vi "Generate Waveform.vi"(0 "signal configuration":refnum<class "SV MLS.lvclass">, 5 "template waveform":waveform(dbl), 9 "block duration (s)":i32, 11 "error in (no error)":errorcluster) -> (4 "signal configuration":refnum<class "SV MLS.lvclass">, 6 "output waveform":waveform(dbl), 10 "samples":i32, 15 "error out":errorcluster)   [LabVIEW 2017, in "SV MLS.lvclass"]
uses:
  <vilib>/addons/_NISVFA/_Generation/Signal Generation/SV MLS/SV MLS.lvclass
  C:/Program Files (x86)/National Instruments/LabVIEW 2017/vi.lib/addons/_NISVFA/_Generation/Signal Generation/SV Signal/SV Signal.lvclass
  <vilib>/addons/_NISVFA/_Generation/Signal Generation/SV Signal/SV Signal.lvclass/SV Signal.ctl
  <vilib>/addons/_NISVFA/_Generation/Signal Generation/SV MLS/SV MLS.lvclass/SV MLS.ctl
  <vilib>/Analysis/NI_AALBase.lvlib
  <vilib>/addons/_NISVFA/_Generation/Signal Generation/SV Signal/SV Signal.lvclass
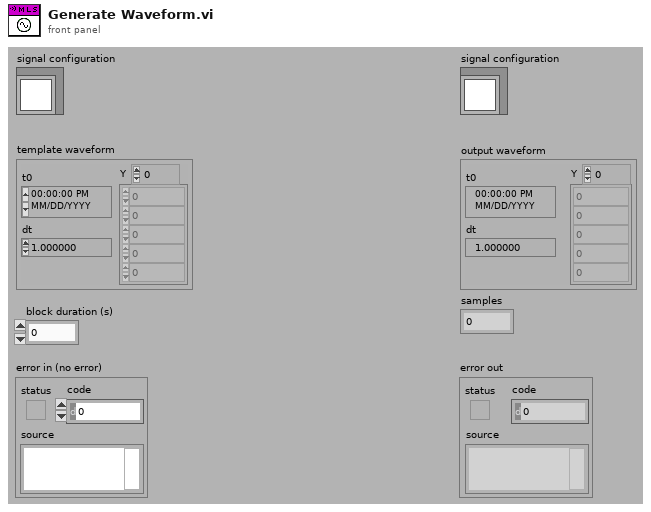
[diagram p1: front panel]
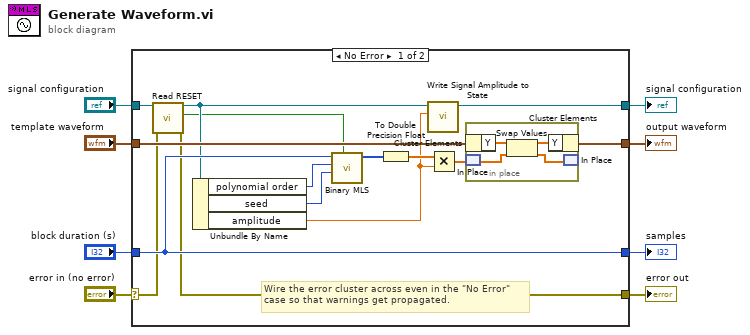
[diagram p0: block diagram]
diagram:
  n1 = case shown="No Error" "error in (no error)" {
    selector: "error in (no error)" -> [w10 w30]
    tunnel: [w9 w30] -> w7
    tunnel: [w15 w29] -> w5
    tunnel: "signal configuration" -> [w13 w29]
    tunnel: [w23 w28] -> w4
    tunnel: [w16 _] -> w3
    tunnel: "block duration (s)" -> [w16 _]
    tunnel: "template waveform" -> [w17 w28]
    frame No Error {
      # "Wire the error cluster across even in the \"No Error\"\ncase so that warnings get propagated."
      n2 = call <vilib>:"Read RESET.vi"("error in (no error)"=w10, "SV Signal in"=w13) -> ("error out"=w9:errorcluster, "RESET"=w11:bool, "SV Signal out"=w12:refnum<class "SV MLS.lvclass">)  [unwired: 7 in]
      n3 = Unbundle By Name(w12) -> ("polynomial order"=w22:i32, "seed"=w21:i64, "amplitude"=w14:dbl)
      n4 = call <vilib>:"Binary MLS.vi"("initialize?"=w11, "seed"=w21, "polynomial order"=w22, "samples"=w16) -> ("mls sequence"=w20:u8[])  [unwired: 6 in, 1 out]
      n5 = To Double Precision Float(number=w20) -> (double precision float=w19:dbl[])
      n6 = call <vilib>:"Write Signal Amplitude to State.vi"("amplitude"=w14, "SV Signal in"=w12) -> ("SV Signal out"=w15:refnum<class "SV MLS.lvclass">)  [unwired: 8 in, 1 out]
      n7 = Multiply(x=w19, y=w14) -> (x*y=w18:dbl[])
      n8 = in-place {
        n9 = in-place-cluster #1(w17) -> ("Y"=w27:dbl[])
        n10 = in-place-match #2(w18) -> (w25:dbl[])
        n11 = Swap Values(12:w27, 14:w25) -> (1:w26:dbl[], 3:w24:dbl[])  [unwired: 1 in]
        n12 = in-place-cluster #1("Y"=w26) -> (w23:waveform(dbl))
        n13 = in-place-match #2(w24) -> ()  [unwired: 1 out]
      }
    }
    frame Error {
    }
  }
  "error out" <- w7
  "signal configuration" <- w5
  "output waveform" <- w4
  "samples" <- w3
